vi "latch.vi"() -> ()   [LabVIEW 2019]
uses:
  5f7d8bd6-e144-4a4a-8e6a-e230b519e0f8.vi
panel:
  in  "stop":bool
  in  "Button":bool
  out "latch":bool
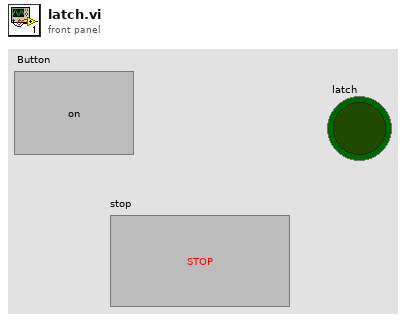
[diagram p1: front panel]
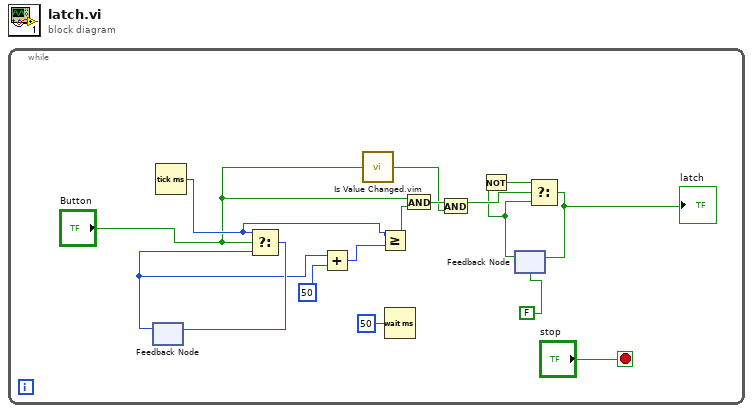
[diagram p0: block diagram]
diagram:
  n1 = while {
    stop <- "stop" stop-if-true
    n2 = feedback #1() -> (w1:u32)  [unwired: 1 in]
    n3 = Tick Count (ms)() -> (millisecond timer value=w13:u32)
    n4 = Select(t=w13, s="Button", f=w1) -> (s? t:f=w11:u32)
    n5 = feedback-in #1(w11) -> ()
    n6 = Add(x=w1, y=u32 50) -> (x+y=w12:u32)
    n7 = call "Is Value Changed.vim"("value"="Button") -> ("changed or first call?"=w7:bool)
    n8 = Greater Or Equal?(x=w13, y=w12) -> (x >= y?=w14:bool)
    n9 = Wait (ms)(milliseconds to wait=u32 50) -> ()  [unwired: 1 out]
    n10 = And(x="Button", y=w14) -> (x .and. y?=w16:bool)
    n11 = And(x=w16, y=w7) -> (x .and. y?=w6:bool)
    n12 = feedback #2(FALSE) -> (w5:bool)
    n13 = Not(x=w5) -> (.not. x?=w2:bool)
    n14 = Select(t=w2, s=w6, f=w5) -> (s? t:f=w3:bool)
    "latch" <- w3
    n15 = feedback-in #2(w3) -> ()
  }
